vi "Act Switch Frame.vi"(8 "error in (no error)":errorcluster, 10 "Frame Num":u32, 11 "LF2R IDE in":refnum<class "LF2R IDE.lvclass">) -> (0 "error out":errorcluster, 3 "LF2R IDE out":refnum<class "LF2R IDE.lvclass">)   [LabVIEW 2018, in "LF2R IDE.lvlib" / "LF2R IDE.lvclass"]
uses:
  LF2R IDE.lvclass
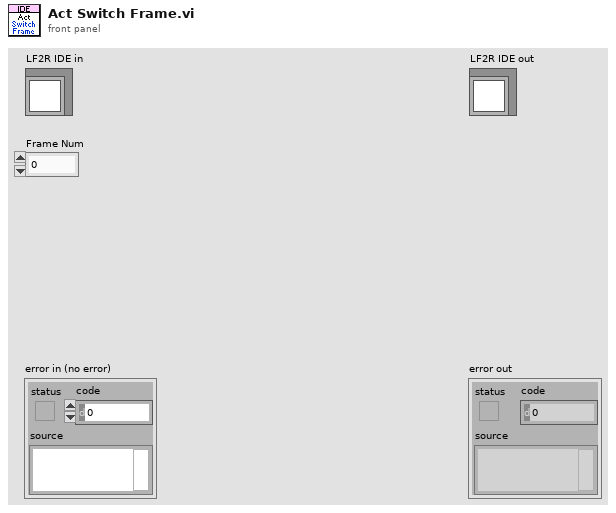
[diagram p1: front panel]
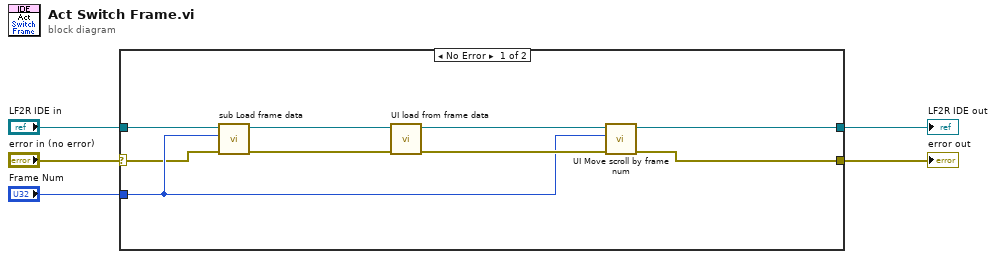
[diagram p0: block diagram]
diagram:
  n1 = case shown="No Error" "error in (no error)" {
    selector: "error in (no error)" -> [w6 w16]
    tunnel: [w12 w16] -> w3
    tunnel: [w13 w15] -> w4
    tunnel: "LF2R IDE in" -> [w14 w15]
    tunnel: "Frame Num" -> [w7 _]
    frame No Error {
      n2 = call "sub Load frame data.vi"("error in (no error)"=w6, "frame number"=w7, "IDE simple in"=w14) -> ("error out"=w10:errorcluster, "IDE simple out"=w11:refnum<class "LF2R IDE.lvclass">)  [unwired: 7 in]
      n3 = call "UI load from frame data.vi"("error in (no error)"=w10, "IDE simple in"=w11) -> ("error out"=w8:errorcluster, "IDE simple out"=w9:refnum<class "LF2R IDE.lvclass">)  [unwired: 8 in]
      n4 = call "UI Move scroll by frame num.vi"("error in (no error)"=w8, "frame number"=w7, "IDE simple in"=w9) -> ("error out"=w12:errorcluster, "IDE simple out"=w13:refnum<class "LF2R IDE.lvclass">)  [unwired: 7 in]
    }
    frame Error {
    }
  }
  "error out" <- w3
  "LF2R IDE out" <- w4
